vi "ModRegistered.vi"(8 "error in (no error)":errorcluster, 11 "JQMHStartup in":refnum<class "ModuleStartup.lvclass">) -> (0 "error out":errorcluster)   [LabVIEW 2024, in "ModuleStartup.lvclass"]
uses:
  ModuleStartup.lvclass
  ModuleStartup.lvclass/ModuleStartup.ctl
  Command.ctl
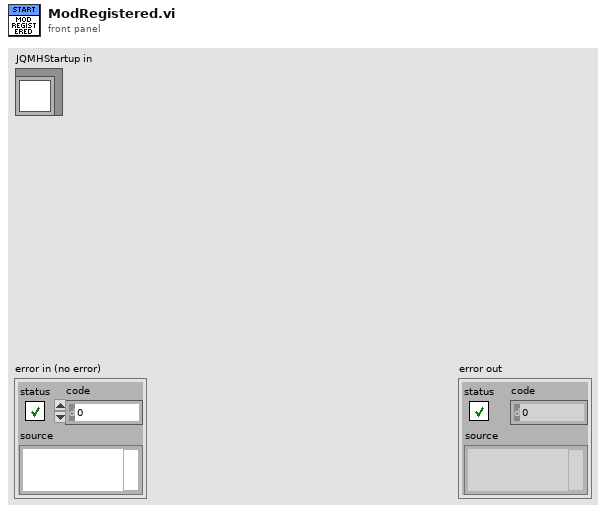
[diagram p1: front panel]
types:
  T1 = typedef "ModuleStartup.lvclass/Command.ctl" = enum16{"Default", "No Override", "Error", "ACK Created", "ACK Mod Reg", "ACK Caller Reg"}
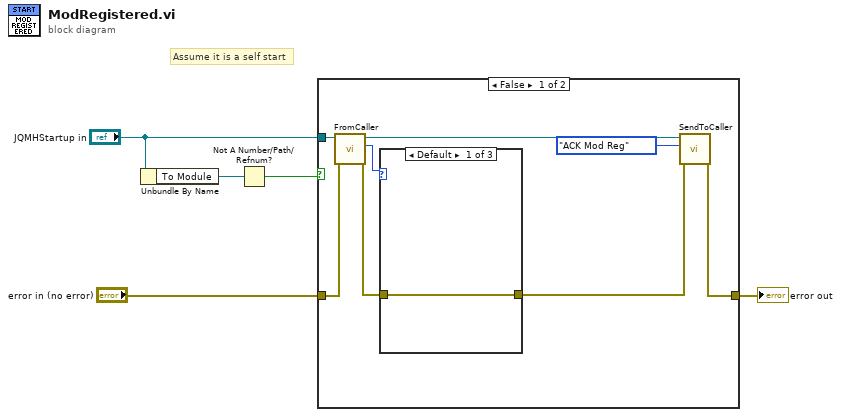
[diagram p0: block diagram]
diagram:
  # "Assume it is a self start"
  n1 = Unbundle By Name("JQMHStartup in") -> ("To Module"=w2:refnum<queue>)
  n2 = Not A Number/Path/Refnum?(number/path/refnum=w2) -> (NaN/Path/Refnum?=w1:bool)
  n3 = case shown="False" w1 {
    tunnel: [w12 w17] -> w5
    tunnel: "error in (no error)" -> [w8 w17]
    tunnel: "JQMHStartup in" -> [w6 _]
    frame False {
      n4 = call "FromCaller.vi"("error in (no error)"=w8, "JQMHStartup in"=w6) -> ("error out"=w10:errorcluster, "Command"=w11:T1, "JQMHStartup out"=w9:refnum<class "ModuleStartup.lvclass">)  [unwired: 6 in, 1 out]
      n5 = case shown="Default" w11 {
        tunnel: [w14 w15 w16] -> w7
        tunnel: w10 -> [w14 w15 w16]
        frame Default {
        }
        frame "Error" {
        }
        frame "ACK Caller Reg" {
        }
      }
      n6 = call "SendToCaller.vi"("error in (no error)"=w7, "Command"=Command."ACK Mod Reg", "JQMHStartup in"=w9) -> ("error out"=w12:errorcluster)  [unwired: 7 in, 1 out]
    }
    frame True {
    }
  }
  "error out" <- w5
